vi "FindDLL.vi"(11 "DLL_Location":path) -> (2 "DLLfilepaths":path[](array[path]), 3 "DLLnames":string[](array[string]))   [LabVIEW 2014]
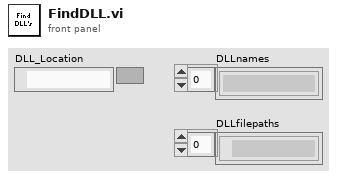
[diagram p1: front panel]
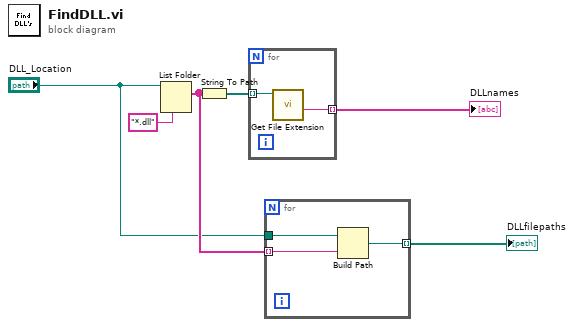
[diagram p0: block diagram]
diagram:
  n1 = List Folder(path="DLL_Location", pattern="*.dll") -> (filenames=w5:string[])  [unwired: 2 in, 3 out]
  n2 = String To Path(string=w5) -> (path=w2:path[])
  n3 = for {
    tunnel: w2 -> [w8] mode=indexing
    tunnel: [w7] -> w3 mode=indexing
    n4 = call <vilib>:"Get File Extension.vi"("file"=w8) -> ("filename without extension"=w7:string)  [unwired: 7 in, 3 out]
  }
  "DLLnames" <- w3
  n5 = for {
    tunnel: "DLL_Location" -> [w11]
    tunnel: w5 -> [w10] mode=indexing
    tunnel: [w9] -> w6 mode=indexing
    n6 = Build Path(base path=w11, name or relative path=w10) -> (appended path=w9:path)
  }
  "DLLfilepaths" <- w6
